vi "P2Y3.vi"() -> ()   [LabVIEW 2020]
panel:
  out "Waveform Graph 2":cluster{i32, i32, dbl[]}[](graph)
  in  "cos amp 2":dbl
  in  "sin amp 2":dbl
  in  "cos sagedus 2":i32
  in  "sin sagedus 2":u32
  in  "Puntkide arv 2":i32
  in  "stop":bool
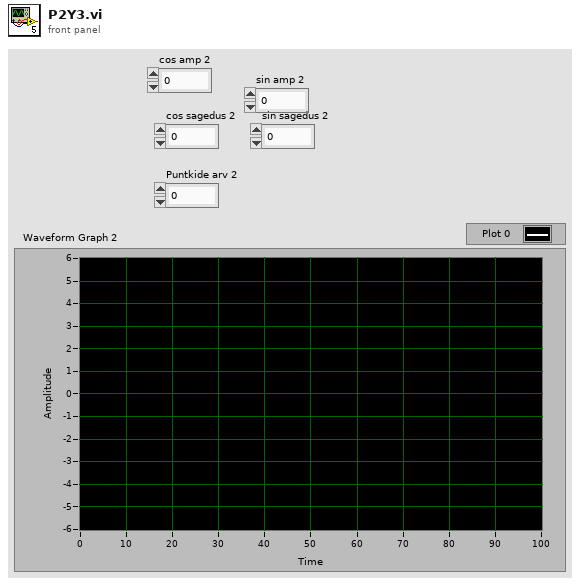
[diagram p1: front panel]
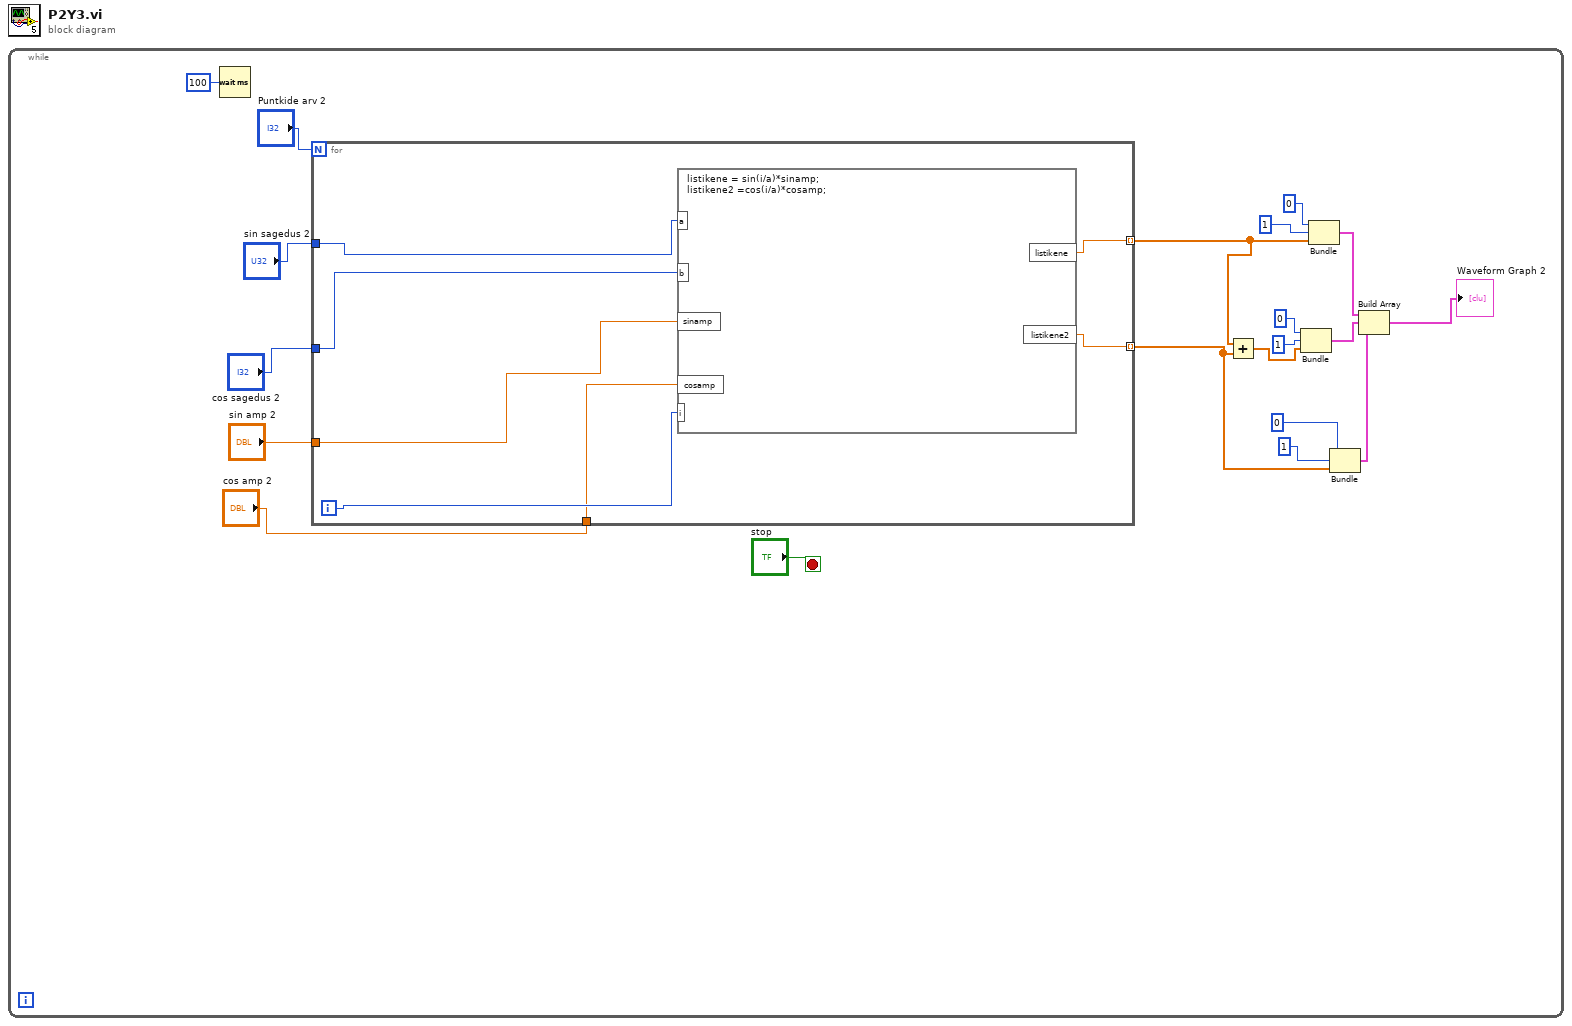
[diagram p0: block diagram]
diagram:
  n1 = while {
    stop <- "stop" stop-if-true
    n2 = Wait (ms)(milliseconds to wait=u32 100) -> ()  [unwired: 1 out]
    n3 = for {
      N: "Puntkide arv 2" -> [_]
      tunnel: "sin sagedus 2" -> [w26]
      tunnel: "cos sagedus 2" -> [w25]
      tunnel: "sin amp 2" -> [w23]
      tunnel: "cos amp 2" -> [w24]
      tunnel: [w22] -> w3 mode=indexing
      tunnel: [w21] -> w2 mode=indexing
      i -> [w27]
      n4 = formula code="listikene = sin(i/a)*sinamp;\nlistikene2 =cos(i/a)*cosamp;"("a"=w26, "b"=w25, "sinamp"=w23, "cosamp"=w24, "i"=w27) -> ("listikene2"=w21:dbl, "listikene"=w22:dbl)
    }
    n5 = Add(x=w3, y=w2) -> (x+y=w9:dbl[])
    n6 = Bundle(0, 1, w9) -> (w6:cluster{i32, i32, dbl[]})  [unwired: 1 in]
    n7 = Bundle(0, 1, w3) -> (w7:cluster{i32, i32, dbl[]})  [unwired: 1 in]
    n8 = Bundle(0, 1, w2) -> (w5:cluster{i32, i32, dbl[]})  [unwired: 1 in]
    n9 = Build Array(w7, w6, w5) -> (→"Waveform Graph 2":cluster{i32, i32, dbl[]}[])
  }
